vi "set_params.vi"(8 "error in (no error)":errorcluster caption="entrée d'erreur (pas d'erreur)", 11 "MultiTaskElasticNetCV.lvclass 2":refnum<class "MultiTaskElasticNetCV.lvclass">) -> (0 "error out":errorcluster caption="sortie d'erreur", 3 "MultiTaskElasticNetCV.lvclass":refnum<class "MultiTaskElasticNetCV.lvclass">)   [LabVIEW 2020, in "MultiTaskElasticNetCV.lvclass"]
uses:
  MultiTaskElasticNetCV.lvclass
  MultiTaskElasticNetCV.lvclass/MultiTaskElasticNetCV.ctl
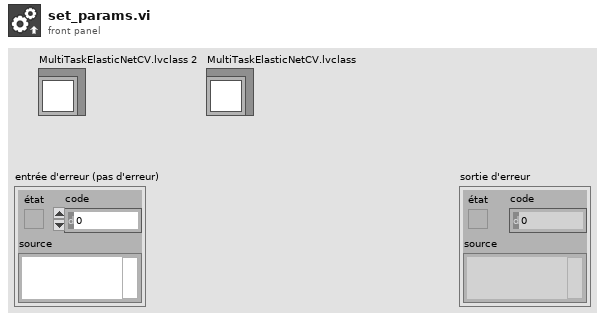
[diagram p1: front panel]
types:
  T1 = typedef "multi_task_elasticnet_cv_params.ctl" = cluster{"l1_ratio":cluster{"l1_ratio_type":string, "l1_ratio_float":dbl, "l1_ratio_list":dbl[]}, "eps":dbl, "n_alphas":dbl, "alphas":cluster{"alphas_type":string, "alphas_list":dbl[]}, "fit_intercept":bool, "normalize":bool, "max_iter":dbl, "tol":dbl, "cv":dbl, "copy_X":bool, "verbose":cluster{"verbose_type":string, "verbose_int":dbl, "verbose_bool":bool}, "n_jobs":dbl, "random_state":dbl, "selection":string}
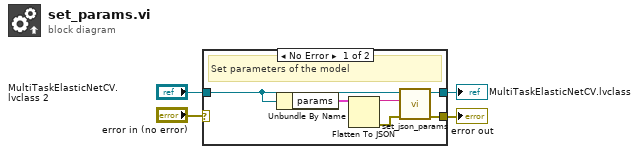
[diagram p0: block diagram]
diagram:
  n1 = case shown="No Error" "error in (no error)" {
    selector: "error in (no error)" -> [_ w12]
    tunnel: [w7 w12] -> w3
    tunnel: [w8 w11] -> w1
    tunnel: "MultiTaskElasticNetCV.lvclass 2" -> [w5 w11]
    frame No Error {
      # "Set parameters of the model"
      n2 = Unbundle By Name(w5) -> ("params"=w10:T1)
      n3 = Flatten To JSON(anything=w10) -> (JSON string=w9:string, 11:w6:errorcluster)  [unwired: 2 in]
      n4 = call-dynamic "set_json_params.vi"("error in (no error)"=w6, "params"=w9, "Model en entrée"=w5) -> ("error out"=w7:errorcluster, "Model en sortie"=w8:refnum<class "MultiTaskElasticNetCV.lvclass">)  [unwired: 7 in]
    }
    frame Error {
    }
  }
  "error out" <- w3
  "MultiTaskElasticNetCV.lvclass" <- w1
